vi "Configure Control Display.vi"(8 "error in (no error)":errorcluster, 11 "Listbox or Tree":refnum<vi>) -> (0 "error out":errorcluster)   [LabVIEW 2011]
doc: "This VI will configure the <b>Listbox or Tree</b> the first time it is called to enable symbols, and set a symbol to allow mixed options for tree controls.\n-------------\nBrian Hoover (hooovahh)"
uses:
  <vilib>/picture/picture.llb/imagedata.ctl
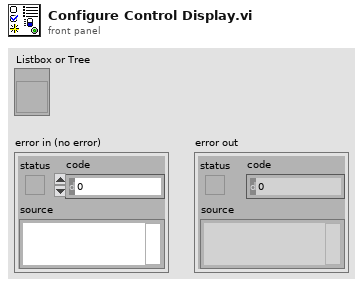
[diagram p1: front panel]
types:
  T1 = typedef "imagedata.ctl" = cluster{"image type":i32, "image depth":i32, "image":u8[], "mask":u8[], "colors":u32[], "Rectangle":cluster{"left":i16, "top":i16, "right":i16, "bottom":i16}}
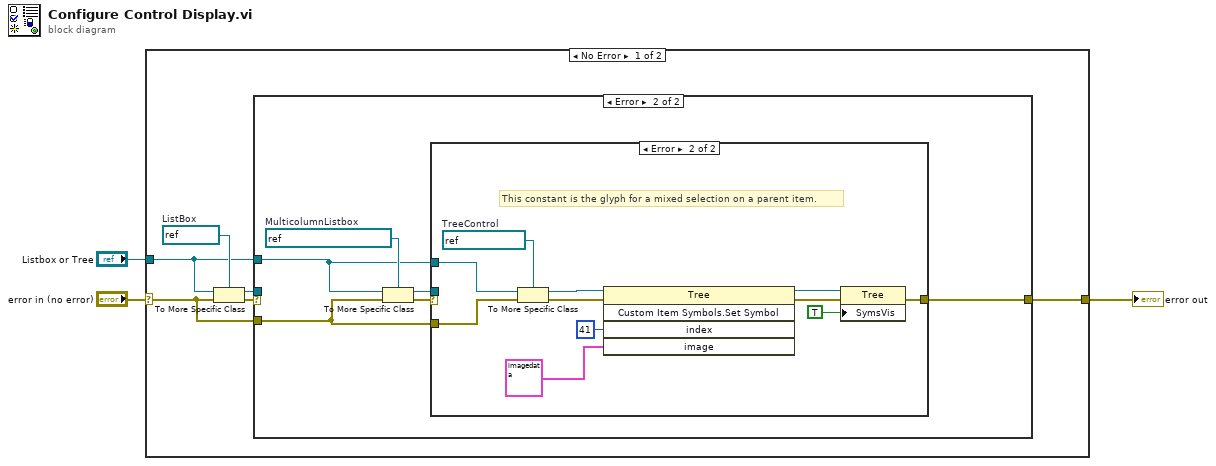
[diagram p0: block diagram]
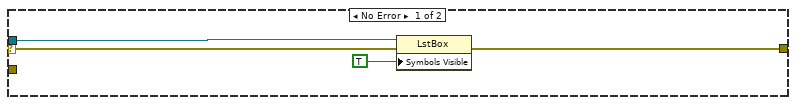
[diagram p2: hidden frame]
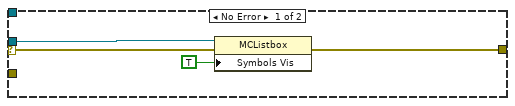
[diagram p3: hidden frame]
diagram:
  n1 = case shown="No Error" "error in (no error)" {
    selector: "error in (no error)" -> [w6 w35]
    tunnel: [w4 w35] -> w2
    tunnel: "Listbox or Tree" -> [w5 _]
    frame No Error {
      w9 = refnum<vi> refnum  # ListBox
      n2 = To More Specific Class(target class=w9, reference=w5, error in=w6) -> (specific class reference=w7:refnum<vi>, error out=w8:errorcluster)
      n3 = case shown="Error" w8 {
        selector: w8 -> [w11 _]
        tunnel: w7 -> [w12 _]
        tunnel: w6 -> [_ w15]
        tunnel: w5 -> [_ w16]
        tunnel: [w10 w14] -> w4
        frame No Error {
          n4 = property class="LstBox"(reference=w12, error in=w11, "Symbols Visible"=TRUE ("Visible Items:Symbols Visible")) -> (error out=w10:errorcluster)  [unwired: 1 out]
        }
        frame Error {
          w19 = refnum<vi> refnum  # MulticolumnListbox
          n5 = To More Specific Class(target class=w19, reference=w16, error in=w15) -> (specific class reference=w17:refnum<vi>, error out=w18:errorcluster)
          n6 = case shown="Error" w18 {
            selector: w18 -> [w21 _]
            tunnel: w17 -> [w22 _]
            tunnel: w16 -> [_ w33]
            tunnel: w15 -> [_ w32]
            tunnel: [w20 w25] -> w14
            frame No Error {
              n7 = property class="MCListbox"(reference=w22, error in=w21, "Symbols Vis"=TRUE ("Visible Items:Symbols Visible")) -> (error out=w20:errorcluster)  [unwired: 1 out]
            }
            frame Error {
              w34 = refnum<vi> refnum  # TreeControl
              # "This constant is the glyph for a mixed selection on a parent item."
              n8 = To More Specific Class(target class=w34, reference=w33, error in=w32) -> (specific class reference=w31:refnum<vi>, error out=w28:errorcluster)
              n9 = invoke class="Tree" method="Custom Item Symbols.Set Symbol"(reference=w31, error in=w28, "index"=41 ("Index"), "image"=T1 {"image type"=0, "image depth"=24, "image"=[142, 143, 143, 142, 143, 143, 142, 143, 143, 142, 143, 143, 142, 143, 143, 142, 143, 143, 142, 143, 143, 142, 143, 143, 142, 143, 143, 142, 143, 143, 142, 143, 143, 142, 143, 143, 142, 143, 143, 142, 143, 143, 244, 244, 244, 244, 244, 244, 244, 244, 244, 244, 244, 244, 244, 244, 244, 244, 244, 244, 244, 244, 244, 244, 244, 244, 244, 244, 244, 244, 244, 244, 244, 244, 244, 142, 143, 143, 142, 143, 143, 244, 244, 244, 41, 98, 141, 42, 98, 142, 42, 98, 142, 42, 98, 141, 41, 97, 140, 40, 96, 138, 40, 94, 135, 39, 91, 132, 38, 89, 128, 244, 244, 244, 142, 143, 143, 142, 143, 143, 244, 244, 244, 41, 98, 141, 127, 200, 228, 123, 195, 225, 117, 190, 221, 110, 183, 217, 104, 175, 211, 96, 167, 204, 89, 157, 196, 36, 86, 124, 244, 244, 244, 142, 143, 143, 142, 143, 143, 244, 244, 244, 41, 97, 139, 123, 194, 224, 47, 168, 213, 47, 166, 211, 46, 164, 208, 45, 159, 203, 43, 153, 197, 80, 146, 187, 35, 82, 118, 244, 244, 244, 142, 143, 143, 142, 143, 143, 244, 244, 244, 40, 95, 137, 116, 187, 218, 46, 164, 209, 45, 162, 206, 44, 157, 201, 43, 151, 194, 41, 145, 187, 71, 134, 177, 32, 76, 110, 244, 244, 244, 142, 143, 143, 142, 143, 143, 244, 244, 244, 39, 93, 133, 109, 179, 212, 44, 158, 201, 43, 153, 196, 42, 147, 190, 40, 141, 183, 37, 133, 174, 62, 121, 166, 30, 70, 101, 244, 244, 244, 142, 143, 143, 142, 143, 143, 244, 244, 244, 38, 90, 129, 102, 169, 203, 42, 148, 191, 40, 142, 184, 38, 135, 176, 36, 127, 167, 34, 119, 159, 52, 107, 154, 27, 64, 92, 244, 244, 244, 142, 143, 143, 142, 143, 143, 244, 244, 244, 36, 85, 123, 93, 157, 194, 39, 137, 179, 36, 129, 170, 34, 120, 160, 31, 111, 150, 30, 105, 143, 44, 96, 143, 25, 59, 85, 244, 244, 244, 142, 143, 143, 142, 143, 143, 244, 244, 244, 35, 81, 117, 85, 146, 184, 76, 134, 174, 68, 122, 164, 59, 110, 153, 50, 101, 147, 44, 95, 143, 37, 89, 140, 25, 59, 85, 244, 244, 244, 142, 143, 143, 142, 143, 143, 244, 244, 244, 33, 78, 113, 31, 73, 106, 29, 68, 97, 26, 62, 89, 25, 59, 85, 25, 59, 85, 25, 58, 85, 25, 58, 85, 25, 59, 85, 244, 244, 244, 142, 143, 143, 142, 143, 143, 244, 244, 244, 244, 244, 244, 244, 244, 244, 244, 244, 244, 244, 244, 244, 244, 244, 244, 244, 244, 244, 244, 244, 244, 244, 244, 244, 244, 244, 244, 244, 244, 244, 142, 143, 143, 142, 143, 143, 142, 143, 143, 142, 143, 143, 142, 143, 143, 142, 143, 143, 142, 143, 143, 142, 143, 143, 142, 143, 143, 142, 143, 143, 142, 143, 143, 142, 143, 143, 142, 143, 143, 142, 143, 143], "mask"=[], "colors"=[], "Rectangle"={"left"=0, "top"=0, "right"=13, "bottom"=13}} ("image data")) -> (reference out=w27:refnum<vi>, error out=w26:errorcluster)  [unwired: 1 in, 3 out]
              n10 = property class="Tree"(reference=w27, error in=w26, "SymsVis"=TRUE ("Visible Items:Symbols Visible")) -> (error out=w25:errorcluster)  [unwired: 1 out]
            }
          }
        }
      }
    }
    frame Error {
    }
  }
  "error out" <- w2
